vi "RT-Main.vi"() -> ()   [LabVIEW 2016]
uses:
  Array AE Data.ctl
  AE Data.ctl
  <vilib>/NI_Real-Time Target Support.lvlib
panel:
  out "Array of AEs":T1=[{"Name"="Peng", "Go?"=TRUE, "Which batch?"=enum."Anything"}, {"Name"="Xue Sheng", "Go?"=TRUE, "Which batch?"=enum."Anything"}, {"Name"="Denny", "Go?"=TRUE, "Which batch?"=enum."Anything"}, {"Name"="Wilbur", "Go?"=TRUE, "Which batch?"=enum."Anything"}, {"Name"="Hafiz", "Go?"=TRUE, "Which batch?"=enum."Anything"}, {"Name"="James", "Go?"=TRUE, "Which batch?"=enum."Anything"}, {"Name"="Sharath", "Go?"=TRUE, "Which batch?"=enum."Anything"}, {"Name"="Habib", "Go?"=TRUE, "Which batch?"=enum."Anything"}, {"Name"="Stephen", "Go?"=TRUE, "Which batch?"=enum."Anything"}]
  in  "Stop Button":bool
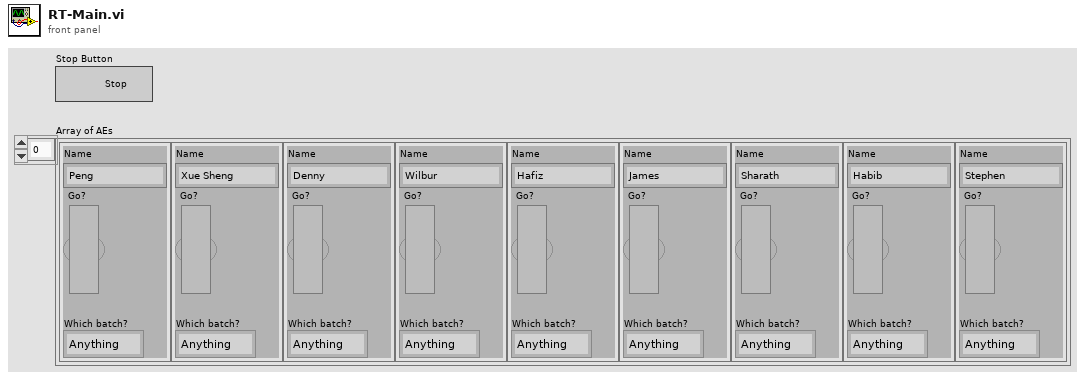
[diagram p1: front panel]
types:
  T1 = typedef "Array AE Data.ctl" = T2[]
  T2 = typedef "AE Data.ctl" = cluster{"Name":string, "Go?":bool, "Which batch?":enum16{"Anything", "First", "Second"}}
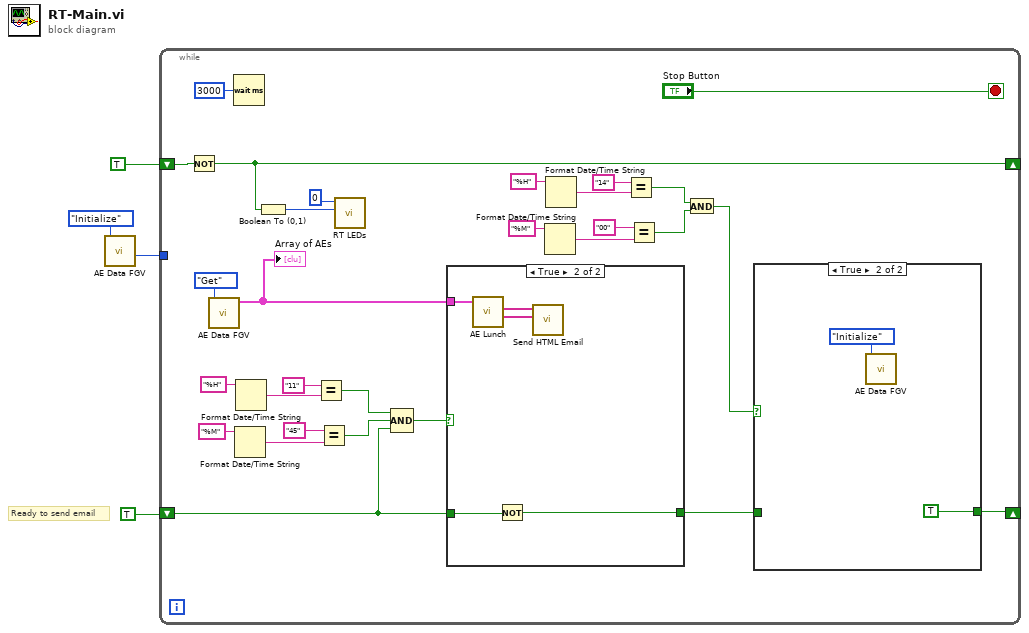
[diagram p0: block diagram]
diagram:
  # "Ready to send email"
  n1 = call "AE Data FGV.vi"("Command"=enum16{"Initialize", "Update", "Get"}."Initialize") -> ("Index"=w2:i32)  [unwired: 9 in, 1 out]
  n2 = while {
    shift-right: [w31] -> _
    shift-left: TRUE -> [w32]
    tunnel: w2 -> [_]
    shift-right: [w5] -> _
    shift-left: TRUE -> [w16]
    stop <- "Stop Button" stop-if-true
    n3 = Not(x=w32) -> (.not. x?=w31:bool)
    n4 = call "AE Data FGV.vi"("Command"=enum16{"Initialize", "Update", "Get"}."Get") -> ("Array of AEs"=w17:T1)  [unwired: 9 in, 1 out]
    "Array of AEs" <- w17
    n5 = Wait (ms)(milliseconds to wait=u32 3000) -> ()  [unwired: 1 out]
    n6 = Format Date/Time String(time format string (%c)="%M") -> (date/time string=w22:string)  [unwired: 2 in]
    n7 = Format Date/Time String(time format string (%c)="%H") -> (date/time string=w24:string)  [unwired: 2 in]
    n8 = Boolean To (0,1)(Boolean=w31) -> (0, 1=w30:i16)
    n9 = Equal?(x="11", y=w24) -> (x = y?=w20:bool)
    n10 = Equal?(x="45", y=w22) -> (x = y?=w19:bool)
    n11 = call <vilib>:"RT LEDs.vi"("State"=w30, "LED Num"=0) -> ()  [unwired: 4 in, 2 out]
    n12 = Compound Arithmetic op=AND(w20, w19, w16) -> (w18:bool)
    n13 = case shown="True" w18 {
      tunnel: w17 -> [_ w42]
      tunnel: w16 -> [w37 w41]
      tunnel: [w37 w40] -> w6
      frame False {
      }
      frame True {
        n14 = call "AE Lunch.vi"("Array of AEs"=w42) -> ("Second Batch"=w38:string[], "First Batch"=w39:string[])  [unwired: 8 in, 1 out]
        n15 = Not(x=w41) -> (.not. x?=w40:bool)
        n16 = call "Send HTML Email.vi"("Second Batch"=w38, "First Batch"=w39) -> ()  [unwired: 8 in, 2 out]
      }
    }
    n17 = Format Date/Time String(time format string (%c)="%M") -> (date/time string=w14:string)  [unwired: 2 in]
    n18 = Format Date/Time String(time format string (%c)="%H") -> (date/time string=w12:string)  [unwired: 2 in]
    n19 = Equal?(x="14", y=w12) -> (x = y?=w9:bool)
    n20 = Equal?(x="00", y=w14) -> (x = y?=w8:bool)
    n21 = And(x=w9, y=w8) -> (x .and. y?=w7:bool)
    n22 = case shown="True" w7 {
      tunnel: w6 -> [w34 _]
      tunnel: [w34 TRUE] -> w5
      frame False {
      }
      frame True {
        n23 = call "AE Data FGV.vi"("Command"=enum16{"Initialize", "Update", "Get"}."Initialize") -> ()  [unwired: 9 in, 2 out]
      }
    }
  }
